vi "Analogue_output.vi"() -> ()   [LabVIEW 2017]
uses:
  <vilib>/rvi/Analysis/common/FxpNativeNode/niFpgaFxpNative.xnode
panel:
  in  "occurrence":refnum<k4>
  in  "Stop index":i16
  in  "Start index":i16
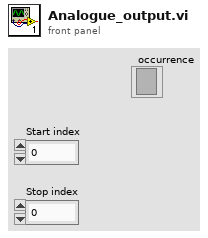
[diagram p1: front panel]
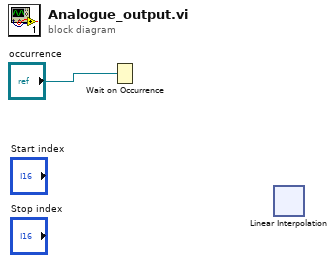
[diagram p0: block diagram]
diagram:
  n1 = Wait on Occurrence(2:"occurrence") -> ()  [unwired: 2 in, 1 out]
  n2 = xnode ("Linear Interpolation")() -> ()  [unwired: 3 in, 1 out]
